vi "Recovery_File_Path.vi"() -> (2 "Recovery File Path":path)   [LabVIEW 2024]
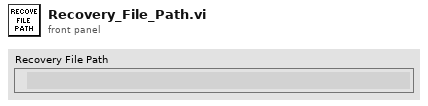
[diagram p1: front panel]
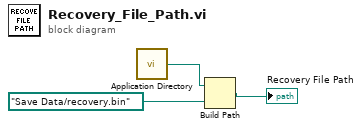
[diagram p0: block diagram]
diagram:
  n1 = call <vilib>:"Application Directory.vi"() -> ("Application Directory"=w3:path)
  n2 = Build Path(base path=w3, name or relative path=path "Save Data/recovery.bin") -> (appended path=→"Recovery File Path":path)
